vi "ClassPanel.vi"(8 "error in (no error)":errorcluster caption="entrée d'erreur (pas d'erreur)", 11 "Triax320.lvclass":refnum<class "Triax320.lvclass">) -> (0 "error out":errorcluster caption="sortie d'erreur", 3 "Triax320.lvclass Out":refnum<class "Triax320.lvclass">)   [LabVIEW 2019, in "Triax320.lvclass"]
uses:
  Triax320.lvclass
  C:/Programmes Labview/LabScanV1A/DevicesClass/BaseDevice/BaseDevice.lvclass
  BaseDevice/Accessor/GetClassEvent.vi
panel:
  in  "Grating":u8(ring) items=["1", "2", "3"]
  out "Moving":bool
  in  "OutSlit":dbl caption="Output Slit (mm)" format="%.3f"
  in  "Stop":bool
  in  "InSlit":dbl caption="Input Slit (mm)" format="%.3f"
  in  "MiseAJour":bool
  in  "Lambda":dbl=60.0 caption="Position(nm)" min=-800.0 max=10000.0 step=0.01 format="%#.3f"
  out "Init Program":bool
  # "Triax 320"
  # "this MUST labeled with class name"
  # "this MUST be present and labeled \"Stop\""
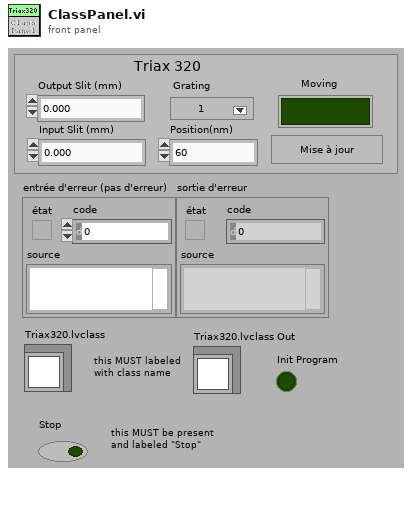
[diagram p1: front panel]
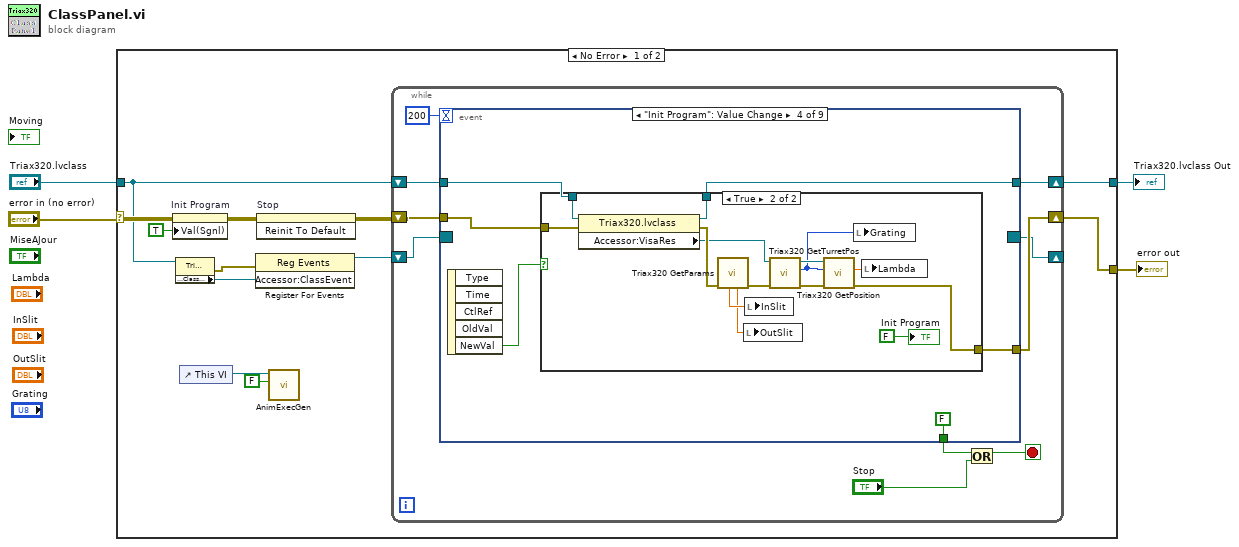
[diagram p0: block diagram]
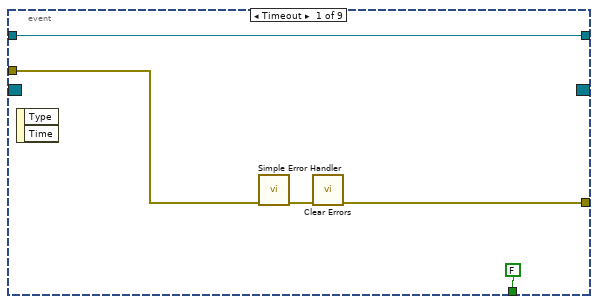
[diagram p2: hidden frame]
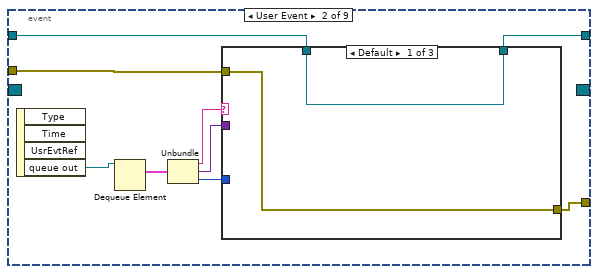
[diagram p3: hidden frame]
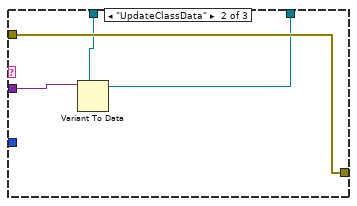
[diagram p4: hidden frame]
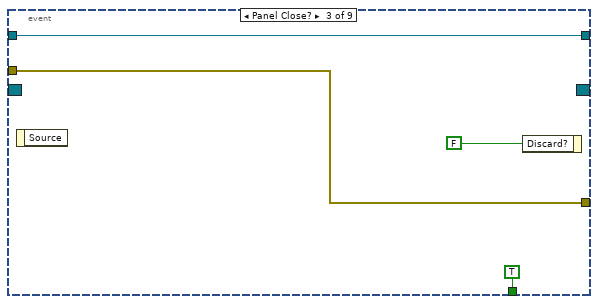
[diagram p6: hidden frame]
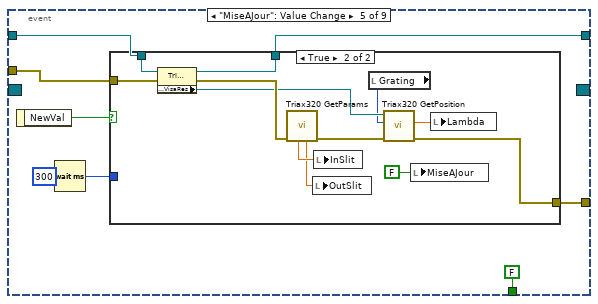
[diagram p8: hidden frame]
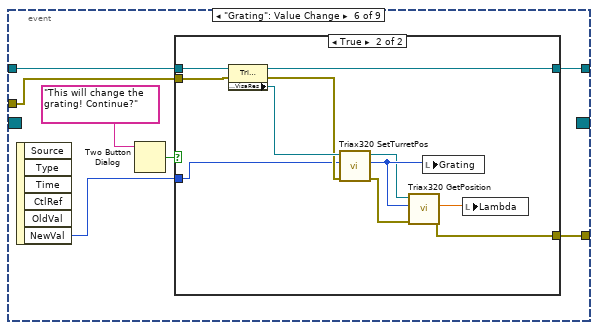
[diagram p10: hidden frame]
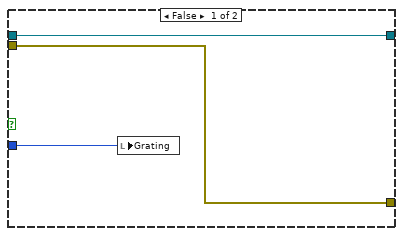
[diagram p11: hidden frame]
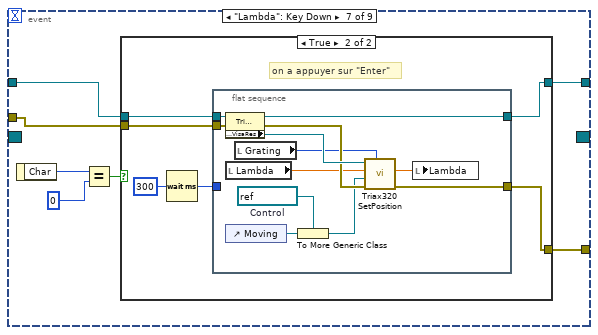
[diagram p12: hidden frame]
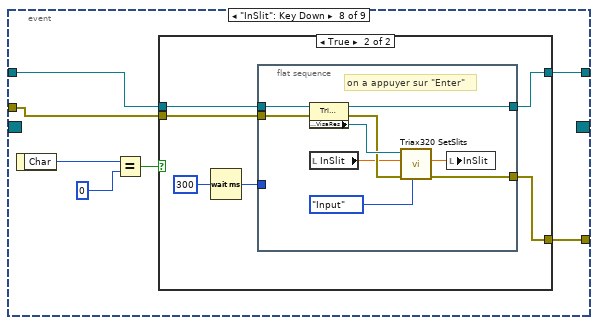
[diagram p14: hidden frame]
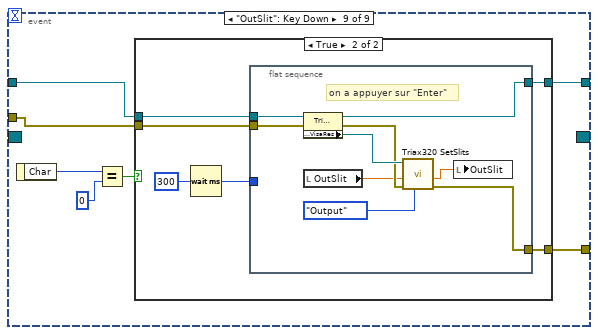
[diagram p16: hidden frame]
diagram:
  n1 = case shown="No Error" "error in (no error)" {
    selector: "error in (no error)" -> [w13 w194]
    tunnel: [w16 w194] -> w3
    tunnel: "Triax320.lvclass" -> [w8 w193]
    tunnel: [w14 w193] -> w1
    frame No Error {
      n2 = property on="Init Program" class="Bool (strict)"(error in=w13, "Val(Sgnl)"=TRUE ("Valeur (Signalisation)")) -> (error out=w12:errorcluster)  [unwired: 1 in, 1 out]
      n3 = property class="Triax320.lvclass"(reference=w8) -> (error out=w10:errorcluster, "Accessor:ClassEvent"=w9:refnum<user-event>)  [unwired: 1 in, 1 out]
      n4 = control-ref of="This VI"() -> (w5:refnum<vi>)
      n5 = register-events(error in=w10, w9) -> (reference out=w7:refnum<event-registration>)  [unwired: 1 in, 1 out]
      n6 = invoke on="Stop" class="Bool (strict)" method="Reinit To Default"(error in=w12) -> (error out=w11:errorcluster)  [unwired: 2 in, 2 out]
      n7 = call <userlib>:"AnimExecGen.vi"("Animer l'exécution ?"=FALSE, "ViRef"=w5) -> ()  [unwired: 9 in, 1 out]
      n8 = while {
        shift-right: [w24] -> w16
        shift-left: w11 -> [w25]
        shift-right: [w21] -> w14
        shift-left: w8 -> [w23]
        shift-right: [w17] -> _
        shift-left: w7 -> [w18]
        stop <- w20 stop-if-true
        n9 = event shown="[3] \"Init Program\": Value Change" {
          selector: w18 -> [_ _ _ _ _ _ _ _ _]
          dyn-events: [_ _ _ _ _ _ _ _ _] -> w17
          timeout: 200 -> [_ _ _ _ _ _ _ _ _]
          tunnel: w25 -> [w29 w39 w50 w57 w81 w99 w120 w147 w172]
          tunnel: [w27 w33 w50 w56 w80 w98 w118 w145 w170] -> w24
          tunnel: w23 -> [w30 w40 w49 w54 w78 w101 w121 w148 w173]
          tunnel: [FALSE _ TRUE FALSE FALSE _ _ _ _] -> w22
          tunnel: [w30 w32 w49 w53 w77 w100 w119 w146 w171] -> w21
          event Timeout {
            n10 = event-data() -> ()  [unwired: 1 in, 2 out]
            n11 = call <vilib>:"Simple Error Handler.vi"("error in (no error)"=w29) -> ("error out"=w28:errorcluster)  [unwired: 4 in, 4 out]
            n12 = call <vilib>:"Clear Errors.vi"("error in (no error)"=w28) -> ("error out"=w27:errorcluster)  [unwired: 5 in, 1 out]
          }
          event User Event {
            n13 = event-data() -> ("queue out"=w37:refnum<queue>)  [unwired: 1 in, 3 out]
            n14 = Dequeue Element(queue=w37) -> (element=w38:cluster{"Message":string, "Data":variant, i32})  [unwired: 2 in, 3 out]
            n15 = Unbundle(w38) -> ("Message"=w36:string, "Data"=w35:variant, w34:i32)
            n16 = case shown="Default" w36 {
              tunnel: w39 -> [w42 w46 w47]
              tunnel: w35 -> [_ w45 _]
              tunnel: w40 -> [w41 w44 w48]
              tunnel: [w41 w43 w48] -> w32
              tunnel: [w42 w46 w47] -> w33
              tunnel: w34 -> [_ _ _]
              frame Default {
              }
              frame "UpdateClassData" {
                n17 = Variant To Data(type=w44, Variant=w45) -> (data=w43:refnum<class "Triax320.lvclass">)  [unwired: 1 in, 1 out]
              }
              frame "MeasDone" {
              }
            }
          }
          event Panel Close? {
            n18 = event-data() -> ()  [unwired: 1 in, 1 out]
            n19 = event-data("Discard?"=FALSE ("Rejeter ?")) -> ()  [unwired: 1 in, 1 out]
          }
          event "Init Program": Value Change {
            n20 = event-data() -> ("NewVal"=w58:bool)  [unwired: 1 in, 4 out]
            n21 = case shown="True" w58 {
              tunnel: w57 -> [w59 w71]
              tunnel: [w59 w66] -> w56
              tunnel: w54 -> [w60 w69]
              tunnel: [w60 w68] -> w53
              frame False {
              }
              frame True {
                n22 = property class="Triax320.lvclass"(reference=w69, error in=w71) -> (reference out=w68:refnum<class "Triax320.lvclass">, error out=w70:errorcluster, "Accessor:VisaRes"=w64:refnum<visa-resource-name>)
                n23 = call <userlib>:"Triax320 GetParams.vi"("error in"=w70) -> ("error out"=w65:errorcluster, "OutSlit"=w72:dbl, "InSlit"=w73:dbl)  [unwired: 5 in, 3 out]
                n24 = local write "OutSlit"(w72) -> ()
                n25 = local write "InSlit"(w73) -> ()
                n26 = call <userlib>:"Triax320 GetTurretPos.vi"("error in (no error)"=w65, "Triax VISA Rsrc"=w64) -> ("error out"=w62:errorcluster, "Grating"=w61:u8, "Triax VISA Rsrc Out"=w63:refnum<visa-resource-name>)  [unwired: 7 in]
                n27 = call <userlib>:"Triax320 GetPosition.vi"("error in (no error)"=w62, "Grating"=w61, "Triax VISA Rsrc"=w63) -> ("error out"=w66:errorcluster, "Lambda Out"=w67:dbl)  [unwired: 6 in, 1 out]
                n28 = local write "Grating"(w61) -> ()
                n29 = local write "Lambda"(w67) -> ()
                "Init Program" <- FALSE
              }
            }
          }
          event "MiseAJour": Value Change {
            n30 = event-data() -> ("NewVal"=w82:bool)  [unwired: 1 in]
            n31 = Wait (ms)(milliseconds to wait=u32 300 ("attente (ms)")) -> (millisecond timer value=w76:u32)
            n32 = case shown="True" w82 {
              tunnel: w81 -> [w83 w93]
              tunnel: [w83 w87] -> w80
              tunnel: w78 -> [w84 w91]
              tunnel: [w84 w90] -> w77
              tunnel: w76 -> [_ _]
              frame False {
              }
              frame True {
                n33 = property class="Triax320.lvclass"(reference=w91, error in=w93) -> (reference out=w90:refnum<class "Triax320.lvclass">, error out=w92:errorcluster, "Accessor:VisaRes"=w89:refnum<visa-resource-name>)
                n34 = call <userlib>:"Triax320 GetParams.vi"("error in"=w92) -> ("error out"=w94:errorcluster, "OutSlit"=w95:dbl, "InSlit"=w96:dbl)  [unwired: 5 in, 3 out]
                n35 = local write "OutSlit"(w95) -> ()
                n36 = local write "InSlit"(w96) -> ()
                n37 = local read "Grating"() -> (w85:u8)
                n38 = call <userlib>:"Triax320 GetPosition.vi"("error in (no error)"=w94, "Grating"=w85, "Triax VISA Rsrc"=w89) -> ("error out"=w87:errorcluster, "Lambda Out"=w88:dbl)  [unwired: 6 in, 1 out]
                n39 = local write "MiseAJour"(FALSE) -> ()
                n40 = local write "Lambda"(w88) -> ()
              }
            }
          }
          event "Grating": Value Change {
            n41 = event-data() -> ("NewVal"=w97:u8)  [unwired: 1 in, 5 out]
            n42 = Two Button Dialog(message="This will change the grating! Continue?") -> (T button?=w102:bool)  [unwired: 2 in]
            n43 = case shown="True" w102 {
              tunnel: w97 -> [w106 w112]
              tunnel: w101 -> [w105 w117]
              tunnel: [w105 w116] -> w100
              tunnel: w99 -> [w104 w114]
              tunnel: [w104 w110] -> w98
              frame False {
                n44 = local write "Grating"(w106) -> ()
              }
              frame True {
                n45 = property class="Triax320.lvclass"(reference=w117, error in=w114) -> (reference out=w116:refnum<class "Triax320.lvclass">, error out=w113:errorcluster, "Accessor:VisaRes"=w115:refnum<visa-resource-name>)
                n46 = call <userlib>:"Triax320 SetTurretPos.vi"("error in (no error)"=w113, "Grating"=w112, "Triax VISA Rsrc"=w115) -> ("error out"=w111:errorcluster, "Grating Out"=w109:u8, "Triax VISA Rsrc Out"=w108:refnum<visa-resource-name>)  [unwired: 6 in]
                n47 = call <userlib>:"Triax320 GetPosition.vi"("error in (no error)"=w111, "Grating"=w109, "Triax VISA Rsrc"=w108) -> ("error out"=w110:errorcluster, "Lambda Out"=w107:dbl)  [unwired: 6 in, 1 out]
                n48 = local write "Grating"(w109) -> ()
                n49 = local write "Lambda"(w107) -> ()
              }
            }
          }
          event "Lambda": Key Down {
            n50 = event-data() -> ("Char"=w124:i16)  [unwired: 1 in]
            n51 = Equal?(x=w124, y=i16 0) -> (x = y?=w122:bool)
            n52 = case shown="True" w122 {
              tunnel: w121 -> [w125 w132]
              tunnel: w120 -> [w126 w131]
              tunnel: [w125 w130] -> w119
              tunnel: [w126 w129] -> w118
              frame False {
              }
              frame True {
                # "on a appuyer sur \"Enter\""
                n53 = Wait (ms)(milliseconds to wait=u32 300 ("attente (ms)")) -> (millisecond timer value=w127:u32)
                n54 = flat-sequence {
                  tunnel: w132 -> [w144]
                  tunnel: w131 -> [w143]
                  tunnel: [w142] -> w130
                  tunnel: [w139] -> w129
                  tunnel: w127 -> [_]
                  frame #0 {
                    w135 = refnum<vi> refnum  # Control
                    n55 = property class="Triax320.lvclass"(reference=w144, error in=w143) -> (reference out=w142:refnum<class "Triax320.lvclass">, error out=w140:errorcluster, "Accessor:VisaRes"=w141:refnum<visa-resource-name>)
                    n56 = local read "Lambda"() -> (w138:dbl)
                    n57 = control-ref of="Moving"() -> (w137:refnum<vi>)
                    n58 = local read "Grating"() -> (w133:u8)
                    n59 = To More Generic Class(target class=w135, reference=w137) -> (generic class reference=w136:refnum<vi>)
                    n60 = call <userlib>:"Triax320 SetPosition.vi"("Grating"=w133, "error in (no error)"=w140, "Refnum Cmde"=w136, "Lambda"=w138, "Triax VISA Rsrc"=w141) -> ("error out"=w139:errorcluster, "Lambda Out"=w134:dbl)  [unwired: 3 in, 2 out]
                    n61 = local write "Lambda"(w134) -> ()
                  }
                }
              }
            }
          }
          event "InSlit": Key Down {
            n62 = event-data() -> ("Char"=w151:i16)  [unwired: 1 in]
            n63 = Equal?(x=w151, y=i16 0) -> (x = y?=w149:bool)
            n64 = case shown="True" w149 {
              tunnel: w148 -> [w152 w159]
              tunnel: w147 -> [w153 w158]
              tunnel: [w152 w157] -> w146
              tunnel: [w153 w156] -> w145
              frame False {
              }
              frame True {
                n65 = Wait (ms)(milliseconds to wait=u32 300 ("attente (ms)")) -> (millisecond timer value=w154:u32)
                n66 = flat-sequence {
                  tunnel: w159 -> [w168]
                  tunnel: w158 -> [w167]
                  tunnel: [w166] -> w157
                  tunnel: [w163] -> w156
                  tunnel: w154 -> [_]
                  frame #0 {
                    # "on a appuyer sur \"Enter\""
                    n67 = property class="Triax320.lvclass"(reference=w168, error in=w167) -> (reference out=w166:refnum<class "Triax320.lvclass">, error out=w164:errorcluster, "Accessor:VisaRes"=w165:refnum<visa-resource-name>)
                    n68 = local read "InSlit"() -> (w162:dbl)
                    n69 = call <userlib>:"Triax320 SetSlits.vi"("Slit"=enum16{"Input", "Output", "Both"}."Input", "error in (no error)"=w164, "InSlit"=w162, "Triax VISA Rsrc"=w165) -> ("error out"=w163:errorcluster, "InSlit Out"=w160:dbl)  [unwired: 4 in, 2 out]
                    n70 = local write "InSlit"(w160) -> ()
                  }
                }
              }
            }
          }
          event "OutSlit": Key Down {
            n71 = event-data() -> ("Char"=w169:i16)  [unwired: 1 in]
            n72 = Equal?(x=w169, y=i16 0) -> (x = y?=w174:bool)
            n73 = case shown="True" w174 {
              tunnel: w173 -> [w176 w183]
              tunnel: w172 -> [w177 w182]
              tunnel: [w176 w181] -> w171
              tunnel: [w177 w180] -> w170
              frame False {
              }
              frame True {
                n74 = Wait (ms)(milliseconds to wait=u32 300 ("attente (ms)")) -> (millisecond timer value=w178:u32)
                n75 = flat-sequence {
                  tunnel: w183 -> [w192]
                  tunnel: w182 -> [w191]
                  tunnel: [w190] -> w181
                  tunnel: [w187] -> w180
                  tunnel: w178 -> [_]
                  frame #0 {
                    # "on a appuyer sur \"Enter\""
                    n76 = property class="Triax320.lvclass"(reference=w192, error in=w191) -> (reference out=w190:refnum<class "Triax320.lvclass">, error out=w188:errorcluster, "Accessor:VisaRes"=w189:refnum<visa-resource-name>)
                    n77 = local read "OutSlit"() -> (w186:dbl)
                    n78 = call <userlib>:"Triax320 SetSlits.vi"("Slit"=enum16{"Input", "Output", "Both"}."Output", "error in (no error)"=w188, "OutSlit"=w186, "Triax VISA Rsrc"=w189) -> ("error out"=w187:errorcluster, "OutSlit Out"=w184:dbl)  [unwired: 4 in, 2 out]
                    n79 = local write "OutSlit"(w184) -> ()
                  }
                }
              }
            }
          }
        }
        n80 = Or(x=w22, y="Stop") -> (x .or. y?=w20:bool)
      }
    }
    frame Error {
    }
  }
  "error out" <- w3
  "Triax320.lvclass Out" <- w1
